vi "LSX Get Command Timeout.vi"(7 "plAtoCalibrate":i32, 8 "error in (no error)":errorcluster, 9 "plAtoMove":i32, 10 "plAtoRead":i32, 11 "lLSID":i32) -> (0 "error out":errorcluster, 1 "plAtoMove out":i32, 2 "plAtoRead out":i32, 3 "function return":i32, 5 "plAtoCalibrate out":i32)   [LabVIEW 2016, in "Tango_DLL.lvlib"]
doc: "TANGOAPI int TANGOCALL LSX_GetCommandTimeout (int lLSID, int *plAtoRead, int *plAtoMove, int *plAtoCalibrate);"
uses:
  Tango_DLL.lvlib
  2017/Microscope Control/Device Library/Stages/Marzhauser/SCAN IM 120 x 80/Tango DLL VIs/Tango_DLL.dll
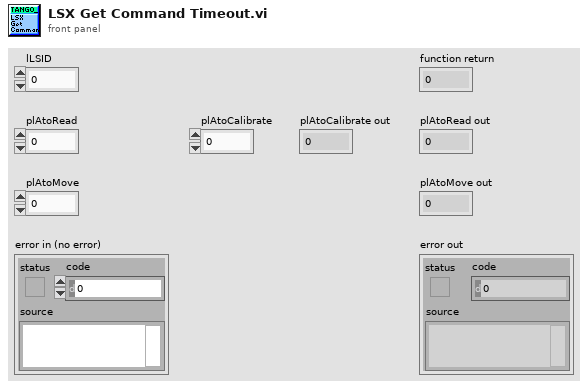
[diagram p1: front panel]
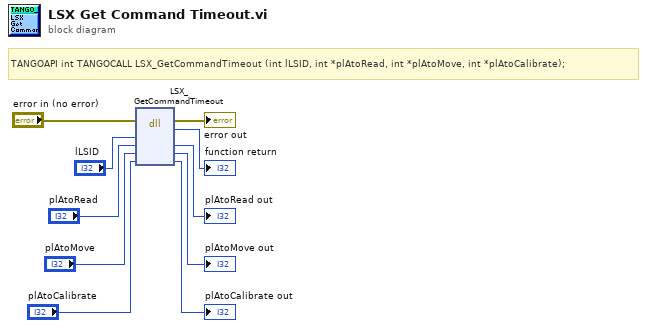
[diagram p0: block diagram]
diagram:
  # "TANGOAPI int TANGOCALL LSX_GetCommandTimeout (int lLSID, int *plAtoRead, int *plAtoMove, int *plAtoCalibrate);"
  n1 = dll-call lib="C:/Users/4PiSMS/Documents/Microscope Control/2017/Microscope Control/Device Library/Stages/Marzhauser/SCAN IM 120 x 80/Tango DLL VIs/Tango_DLL.*" fn="LSX_GetCommandTimeout"(error in="error in (no error)", "lLSID"="lLSID", "plAtoRead"="plAtoRead", "plAtoMove"="plAtoMove", "plAtoCalibrate"="plAtoCalibrate") -> (error out=→"error out":errorcluster, →"function return":i32, "plAtoRead"=→"plAtoRead out":i32, "plAtoMove"=→"plAtoMove out":i32, "plAtoCalibrate"=→"plAtoCalibrate out":i32)  [unwired: 3 in, 1 out]
